vi "average-z-data.vi"(10 "Boolean":bool, 11 "z-data":sgl) -> (2 "MEAN":sgl, 3 "mean is valid":bool)   [LabVIEW 2015]
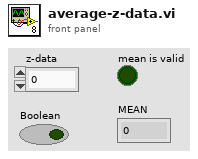
[diagram p1: front panel]
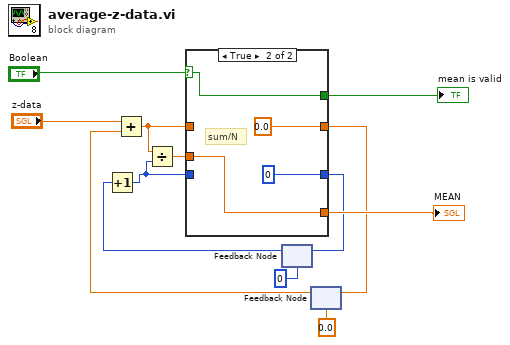
[diagram p0: block diagram]
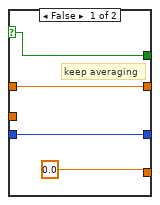
[diagram p2: hidden frame]
diagram:
  n1 = feedback #1(i16 0) -> (w6:i16)
  n2 = Increment(x=w6) -> (x+1=w9:i16)
  n3 = feedback #2(sgl 0.0) -> (w7:sgl)
  n4 = Add(x="z-data", y=w7) -> (x+y=w10:sgl)
  n5 = Divide(x=w10, y=w9) -> (x/y=w11:sgl)
  n6 = case shown="True" "Boolean" {
    selector: "Boolean" -> [w14 w18]
    tunnel: [w15 sgl 0.0] -> w2
    tunnel: [w16 i16 0] -> w3
    tunnel: w9 -> [w16 _]
    tunnel: [sgl 0.0 w19] -> w12
    tunnel: w10 -> [w15 _]
    tunnel: w11 -> [_ w19]
    tunnel: [w14 w18] -> w13
    frame False {
      # "keep averaging"
    }
    frame True {
      # "sum/N"
    }
  }
  "MEAN" <- w12
  "mean is valid" <- w13
  n7 = feedback-in #1(w3) -> ()
  n8 = feedback-in #2(w2) -> ()
